vi "PathPlanner_Path_MirrorTranslation.vi"(11 "inTranslation":T1 {"Y" format="%14.3f"; "X" format="%14.3f"}) -> (3 "MirrorTranslation":T1 {"Y" format="%14.3f"; "X" format="%14.3f"})   [LabVIEW 2019, in "PathPlanner24.lvlib"]
doc: "Get a specific point along this path\n\nInputs: \n - Path - cluster - path definition data structure\n - index - integer - Index of the point to get\n\nOutputs:\n - Point - PathPoint - The point at the given index"
uses:
  PathPlanner24.lvlib
  <vilib>/Rock Robotics/WPI/ThirdParty/JAS_Junk/TrajLib/Trajectory_Library.lvlib
  <vilib>/Rock Robotics/WPI/ThirdParty/JAS_Junk/TrajLib/TypeDef/TRANSLATION2D.ctl
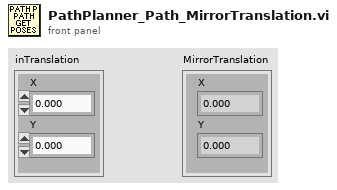
[diagram p1: front panel]
types:
  T1 = typedef "Trajectory_Library.lvlib/TRANSLATION2D.ctl" = cluster{"X":dbl, "Y":dbl}
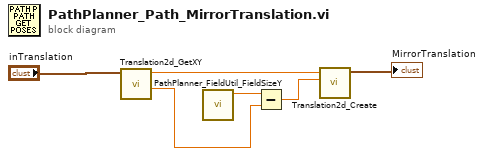
[diagram p0: block diagram]
diagram:
  n1 = call <vilib>:"Translation2d_GetXY.vi"("In Translation"="inTranslation") -> ("Y"=w3:dbl, "X"=w5:dbl)  [unwired: 9 in]
  n2 = call "PathPlanner_FieldUtil_FieldSizeY.vi"() -> ("FieldSizeY_M"=w4:dbl)  [unwired: 11 in]
  n3 = Subtract(x=w4, y=w3) -> (x-y=w2:dbl)
  n4 = call <vilib>:"Translation2d_Create.vi"("Y"=w2, "X"=w5) -> ("TRANSLATION"=→"MirrorTranslation":T1)  [unwired: 9 in]
